vi "DL-Read (TDT).vi"(0 "RPcoX in":refnum<k7>, 7 "Npts":i32, 11 "error in (no error)":errorcluster) -> (4 "RPcoX out":refnum<k7>, 6 "data":waveform(dbl)[](array[waveform]), 15 "error out":errorcluster)   [LabVIEW 2020]
uses:
  epl-vi-lib/PXI DAQ VIs/TDT VIs/TDT-Signal Bank Action.ctl
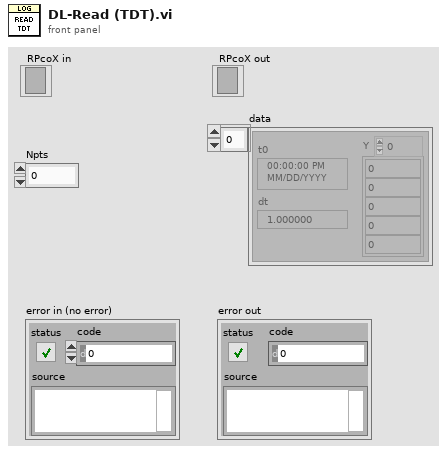
[diagram p1: front panel]
types:
  T1 = typedef "TDT-Signal Bank Action.ctl" = enum16{"Init", "Write", "Read", "Rewrite", "Reset", "Recycle", "Ramp up", "Ramp down", "Zero"}
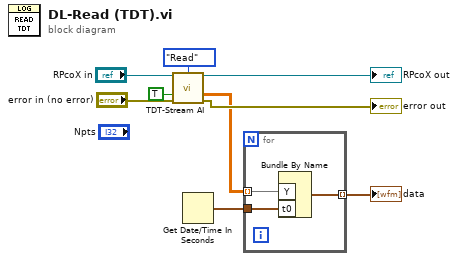
[diagram p0: block diagram]
diagram:
  n1 = call "TDT-Stream AI.vi"("RPcox"="RPcoX in", "Action"=TDT-Signal_Bank_Action."Read", "AI only"=TRUE, "error in (no error)"="error in (no error)") -> ("RPcoX thru"=→"RPcoX out":refnum<k7>, "AI Waveforms"=w4:dbl[][], "error out"=→"error out":errorcluster)  [unwired: 9 in]
  n2 = Get Date/Time In Seconds() -> (seconds since 1Jan1904=w2:timestamp)
  n3 = for {
    tunnel: w4 -> [w12] mode=indexing
    tunnel: [w11] -> w3 mode=indexing
    tunnel: w2 -> [w10]
    n4 = Bundle By Name("Y"=w12, "t0"=w10) -> (w11:waveform(dbl))  [unwired: 1 in]
  }
  "data" <- w3
